vi "PingCmdLine.vi"(8 "error in (no error)":errorcluster, 11 "IP Address":string) -> (0 "error out":errorcluster, 1 "Match?(t)":bool, 2 "Ip_out":string)   [LabVIEW 2018]
panel:
  out "before substring":string
  out "array":string[](array[string])
  out "standard output":string
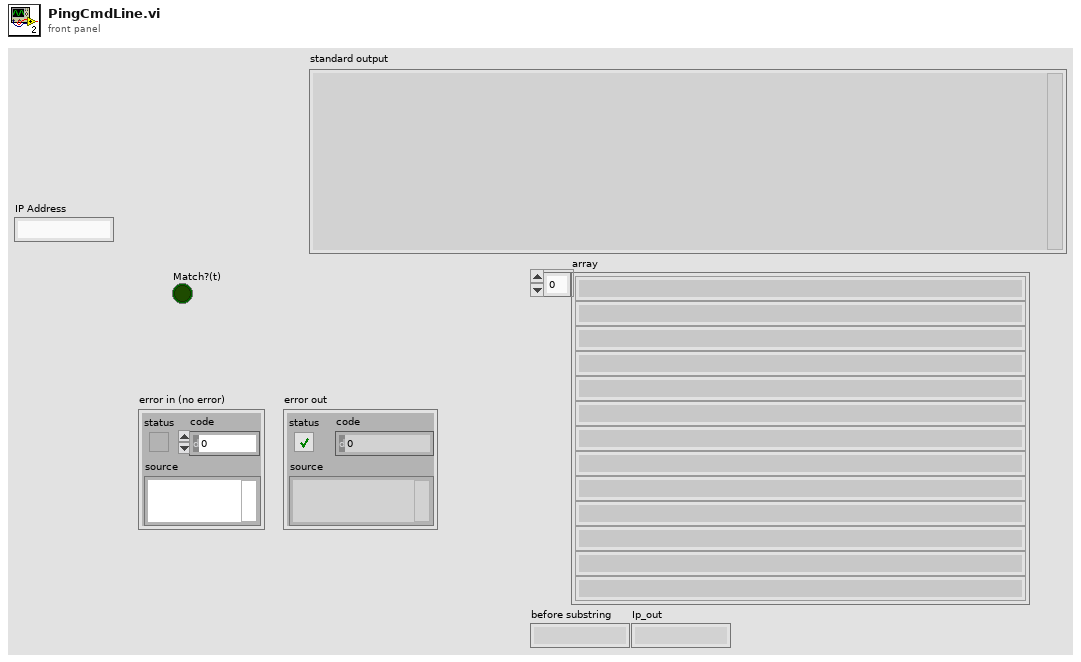
[diagram p1: front panel]
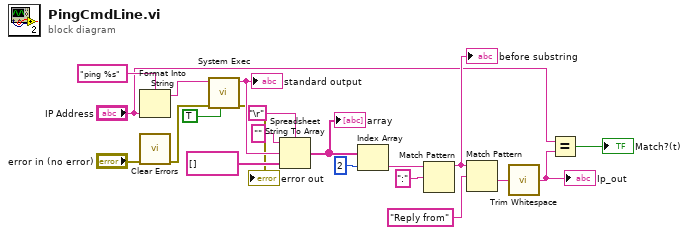
[diagram p0: block diagram]
diagram:
  n1 = Format Into String(format string="ping %s", "IP Address") -> (resulting string=w17:string)  [unwired: 2 in, 1 out]
  n2 = call <vilib>:"Clear Errors.vi"("error in (no error)"="error in (no error)") -> ("error out"=w20:errorcluster)  [unwired: 5 in, 1 out]
  n3 = call <vilib>:"System Exec.vi"("run minimized? (F)"=TRUE, "error in (no error)"=w20, "command line"=w17) -> ("error out"=→"error out":errorcluster, "standard output"=w16:string)  [unwired: 5 in, 2 out]
  "standard output" <- w16
  n4 = Spreadsheet String To Array(delimiter (Tab)="\r", format string="", spreadsheet string=w16, array type (2D Dbl)=string[] []) -> (array=w12:string[])
  "array" <- w12
  n5 = Index Array(array=w12, index=2) -> (element=w10:string)
  n6 = Match Pattern(string=w10, regular expression=":") -> (before substring=w6:string)  [unwired: 1 in, 3 out]
  "before substring" <- w6
  n7 = Match Pattern(string=w6, regular expression="Reply from") -> (after substring=w7:string)  [unwired: 1 in, 3 out]
  n8 = call <vilib>:"Trim Whitespace.vi"("string"=w7) -> ("trimmed string"=w5:string)  [unwired: 1 in]
  "Ip_out" <- w5
  n9 = Equal?(x="IP Address", y=w5) -> (x = y?=→"Match?(t)":bool)
